vi "TDMS.OpenAdvanced.Wait.vi"(8 "error in (no error)":errorcluster, 11 "file path":path) -> (0 "error out":errorcluster, 3 "tdms file out":refnum<k34>)   [LabVIEW 2016]
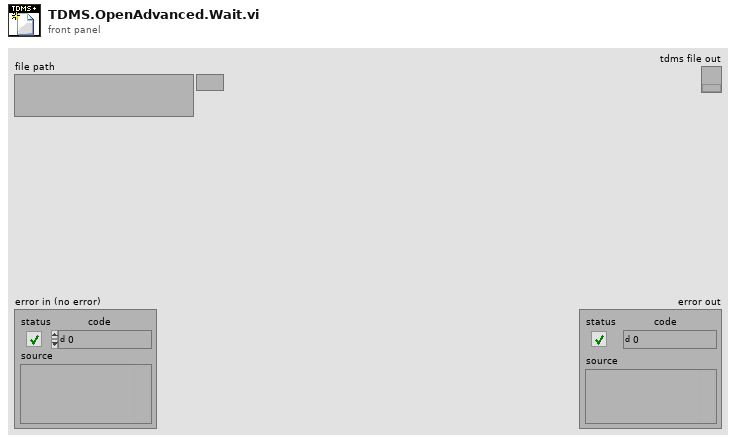
[diagram p1: front panel]
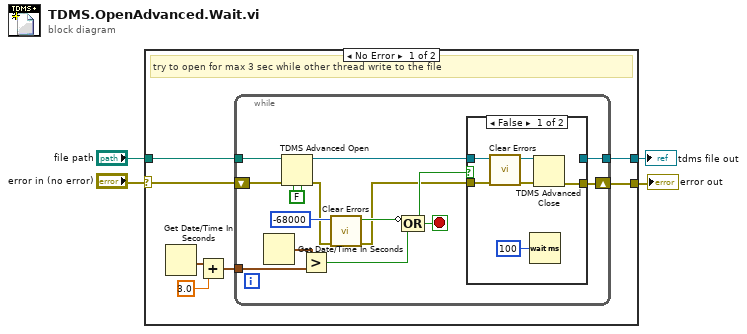
[diagram p0: block diagram]
diagram:
  n1 = case shown="No Error" "error in (no error)" {
    selector: "error in (no error)" -> [w10 w33]
    tunnel: "file path" -> [w11 _]
    tunnel: [w9 _] -> w1
    tunnel: [w5 w33] -> w2
    frame No Error {
      # "try to open for max 3 sec while other thread write to the file"
      n2 = Get Date/Time In Seconds() -> (seconds since 1Jan1904=w7:timestamp)
      n3 = Add(x=w7, y=3.0) -> (x+y=w6:timestamp)
      n4 = while {
        tunnel: w11 -> [w25]
        tunnel: [w21] -> w9
        tunnel: w6 -> [w18]
        shift-right: [w14] -> w5
        shift-left: w10 -> [w24]
        stop <- w17 stop-if-true
        w12 = FALSE ("disable buffering? (T)")
        n5 = Get Date/Time In Seconds() -> (seconds since 1Jan1904=w19:timestamp)
        n6 = TDMS Advanced Open(4:w12, 6:w12, 8:w24, 11:w25) -> (0:w15:errorcluster, 3:w22:refnum<k34>)  [unwired: 1 in, 1 out]
        n7 = Greater?(x=w19, y=w18) -> (0:w16:bool)
        n8 = call <vilib>:"Clear Errors.vi"("error in (no error)"=w15, "specific error code to clear (0: all)"=-68000) -> ("error out"=w13:errorcluster, "specific error cleared?"=w20:bool)  [unwired: 4 in]
        n9 = Compound Arithmetic op=OR(invert w20, w16) -> (w17:bool)
        n10 = case shown="False" w17 {
          tunnel: w22 -> [w30 w32]
          tunnel: [_ w32] -> w21
          tunnel: [w29 w31] -> w14
          tunnel: w13 -> [w28 w31]
          frame False {
            n11 = call <vilib>:"Clear Errors.vi"("error in (no error)"=w28) -> ("error out"=w27:errorcluster)  [unwired: 5 in, 1 out]
            n12 = Wait (ms)(milliseconds to wait=u32 100) -> ()  [unwired: 1 out]
            n13 = TDMS Advanced Close(8:w27, 11:w30) -> (0:w29:errorcluster)  [unwired: 2 in, 1 out]
          }
          frame True {
          }
        }
      }
    }
    frame Error {
    }
  }
  "error out" <- w2
  "tdms file out" <- w1
